vi "Create Path (path).vi"(5 "URI-Component.Path":refnum<class "URI-Component.Path.lvclass">, 8 "error in (no error)":errorcluster, 10 "base-path":string, 11 "Path":path) -> (0 "error out":errorcluster, 1 "Valid":bool, 2 "Path type":T1=enum."path-abempty", 3 "URI-Component.Path":refnum<class "URI-Component.Path.lvclass">)   [LabVIEW 2013, in "openURI.lvlib" / "URI-Component.Path.lvclass"]
uses:
  URI-Component.Path.lvclass
  path type -- enum.ctl
  openURI.lvlib
panel:
  out "common path":string
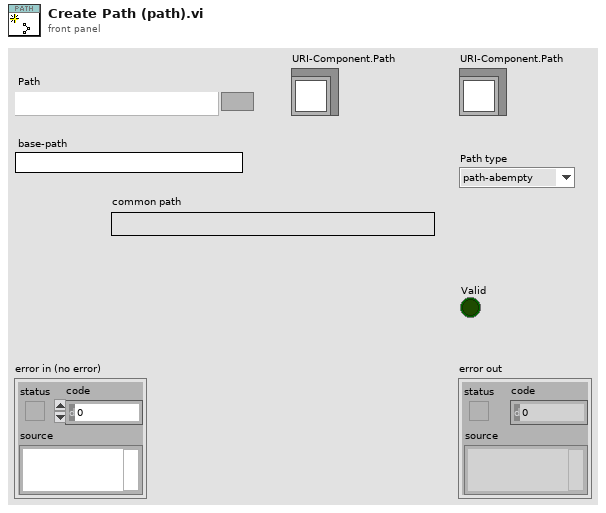
[diagram p1: front panel]
types:
  T1 = typedef "openURI.lvlib/URI-Component.Path.lvclass/path type -- enum.ctl" = enum16{"invalid", "path-abempty", "path-absolute", "path-noscheme", "path-rootless", "path-empty"}
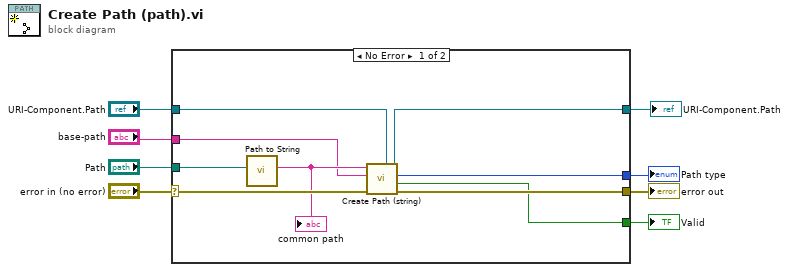
[diagram p0: block diagram]
diagram:
  n1 = case shown="No Error" "error in (no error)" {
    selector: "error in (no error)" -> [w16 w19]
    tunnel: [w15 w19] -> w7
    tunnel: [w9 w18] -> w5
    tunnel: "URI-Component.Path" -> [w17 w18]
    tunnel: [w14 _] -> w4
    tunnel: [w13 _] -> w3
    tunnel: "Path" -> [w12 _]
    tunnel: "base-path" -> [w10 _]
    frame No Error {
      n2 = call "Path to String.vi"("specific path"=w12) -> ("common path"=w11:string)  [unwired: 10 in]
      "common path" <- w11
      n3 = call "Create Path (string).vi"("URI-Component.Path"=w17, "error in (no error)"=w16, "base-path"=w10, "Path"=w11) -> ("error out"=w15:errorcluster, "Valid"=w13:bool, "Path type"=w14:T1, "URI-Component.Path"=w9:refnum<class "URI-Component.Path.lvclass">)  [unwired: 4 in]
    }
    frame Error {
    }
  }
  "error out" <- w7
  "URI-Component.Path" <- w5
  "Path type" <- w4
  "Valid" <- w3
